vi "NewWafer.vi"(2 "error in":errorcluster) -> (3 "Wafer Out":string, 4 "Test Out":string, 5 "Canceled":bool, 6 "error out":errorcluster)   [LabVIEW 2012]
panel:
  in  "Cancel":bool
  in  "Continue":bool
  in  "Test":string(combo)
  in  "Wafer ID":string
  # "Enter Wafer ID and Test Type"
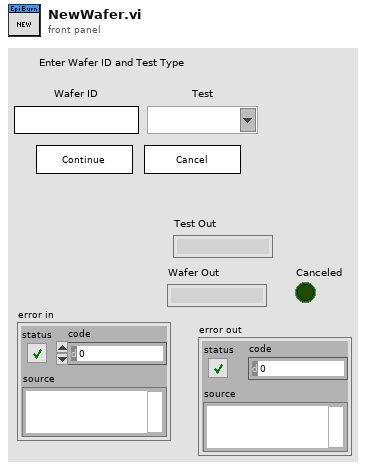
[diagram p1: front panel]
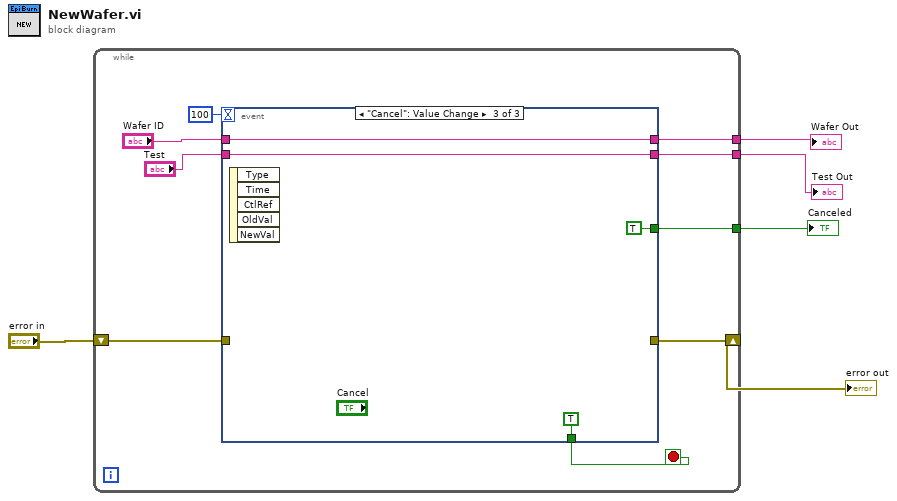
[diagram p0: block diagram]
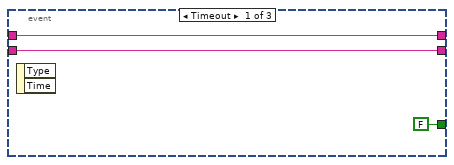
[diagram p2: hidden frame]
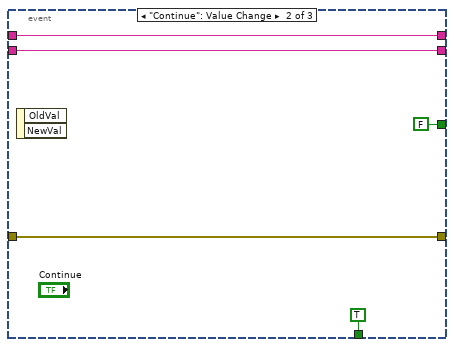
[diagram p3: hidden frame]
diagram:
  n1 = while {
    tunnel: [w11] -> w5
    tunnel: [w10] -> w4
    tunnel: [w9] -> w3
    shift-right: [w7] -> w1
    shift-left: "error in" -> [w6]
    stop <- w12 stop-if-true
    n2 = event shown="[2] \"Cancel\": Value Change" {
      selector: _ -> [_ _ _]
      dyn-events: _ -> [_ _ _]
      timeout: 100 -> [_ _ _]
      tunnel: "Wafer ID" -> [w17 w20 w25]
      tunnel: "Test" -> [w16 w19 w24]
      tunnel: [_ TRUE ("Cancel") TRUE ("Cancel")] -> w12
      tunnel: [FALSE ("Cancel") FALSE ("Cancel") TRUE ("Cancel")] -> w11
      tunnel: [w17 w20 w25] -> w10
      tunnel: [w16 w19 w24] -> w9
      tunnel: [_ w18 _] -> w7
      tunnel: w6 -> [_ w18 _]
      event Timeout {
        n3 = event-data() -> ()  [unwired: 1 in, 2 out]
      }
      event "Continue": Value Change {
        n4 = event-data() -> ()  [unwired: 1 in, 2 out]
      }
      event "Cancel": Value Change {
        n5 = event-data() -> ()  [unwired: 1 in, 5 out]
      }
    }
  }
  "Wafer Out" <- w4
  "Test Out" <- w3
  "Canceled" <- w5
  "error out" <- w1
